vi "Sxx To Dkm.vi"(8 "error in (no error)":errorcluster, 9 "error":i32, 10 "units":i32, 11 "sXx":string) -> (0 "error out":i32, 1 "error out 2":errorcluster, 2 "dkm":dbl, 3 "sXx out":string)   [LabVIEW 2023, in "POSCONV.lvlib"]
doc: "Converts string input to double kilometres by setting the Units Control:\n\n1. case IN_MI:\n2. case IN_KM:\n3. case IN_M:\n4. case IN_ST:\n5. case IN_DMI:\n\ndouble SxxToDkm(char *sXx, int units, int *error);"
uses:
  POSCONV.lvlib
  C:/Users/J Gordon/Documents/Rail Tech/TV-HR/02 - Code/Modules/POSCONV/POSCONV.dll
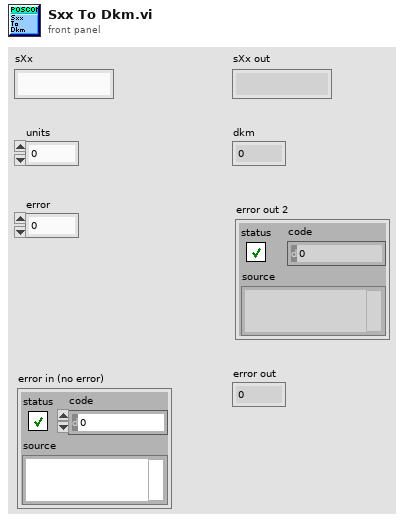
[diagram p1: front panel]
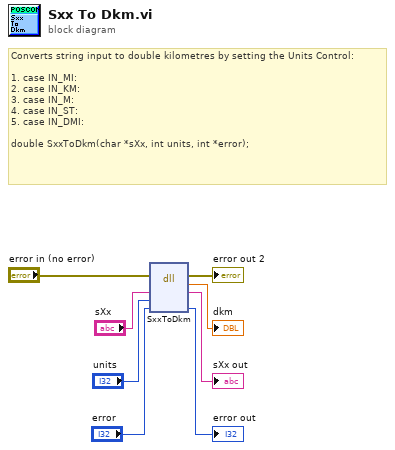
[diagram p0: block diagram]
diagram:
  # "Converts string input to double kilometres by setting the Units Control:\n\n1. case IN_MI:\n2.\tcase IN_KM:\n3.\tcase IN_M:\n4.\tcase IN_ST:\n5.\tcase IN_DMI:\n\ndouble SxxToDkm(char *sXx, int units, int *error);"
  n1 = dll-call lib="C:/Users/J Gordon/Documents/Rail Tech/TV-HR/02 - Code/Modules/POSCONV/POSCONV.*" fn="SxxToDkm"(error in="error in (no error)", "sXx"="sXx", "units"="units", "error"="error") -> (error out=→"error out 2":errorcluster, →"dkm":dbl, "sXx"=→"sXx out":string, "error"=→"error out":i32)  [unwired: 3 in, 1 out]
